vi "Register Disabled Save.vi"(8 "error in (no error)":errorcluster, 11 "UI Controller in":refnum<class "UI Controller.lvclass">) -> (0 "error out":errorcluster, 3 "UI Controller out":refnum<class "UI Controller.lvclass">)   [LabVIEW 2020, in "UI Controller.lvlib" / "UI Controller.lvclass"]
uses:
  UI Controller.lvclass
  C:/Program Files/National Instruments/LabVIEW 2020/vi.lib/ActorFrameworkMVC/Abstract Controller/Abstract Controller/Abstract Controller.lvclass
  Models/Yaml Model/Yaml Model Messages/Register Disabled Save Msg/Register Disabled Save Msg.lvclass
  C:/Program Files/National Instruments/LabVIEW 2020/vi.lib/ActorFramework/Message/Message.lvclass
  Views/Side Menu View/Side Menu View Messages/Concrete Disabled Save Msg/Concrete Disabled Save Msg.lvclass
  C:/Program Files/National Instruments/LabVIEW 2020/vi.lib/ActorFrameworkObserver/Data Message/Data Message.lvclass
  <vilib>/ActorFramework/Message Enqueuer/Message Enqueuer.lvclass/Message Enqueuer.ctl
  Models/Map Model/Map Model Messages/Register Disabled Save Msg/Register Disabled Save Msg.lvclass
  <vilib>/ActorFramework/Message Priority Queue/Priority Enqueue.vi
  <vilib>/ActorFrameworkMVC/Abstract Controller/Abstract Controller/Abstract Controller.lvclass
  <vilib>/ActorFramework/Message Enqueuer/Message Enqueuer.lvclass
panel:
  # "NOTICE -- YOU MUST LEAVE THIS NOTICE IN PLACE.\n\nCopyright (c) 2017, LIANG LIU Shawn.Liu.cn@gmail.com\nAll rights reserved.\n\nRedistribution and use in source and binary forms, with or without modification, are permitted provided that the following conditions are met:\n-Redistributions of source code must retain the above copyright notice, this list of conditions and the following disclaimer.\n-Redistributions in binary form must reproduce the above copyright notice, this list of conditions and the following disclaimer in the documentation and/or other materials provided with the distribution.\n-Neither the name of the eLp nor the names of its contributors may be used to endorse or promote products derived from this software without specific prior written permission.\n\nTHIS SOFTWARE IS PROVIDED BY THE COPYRIGHT HOLDERS AND CONTRIBUTORS \"AS IS\" AND ANY EXPRESS OR IMPLIED WARRANTIES, INCLUDING, BUT NOT LIMITED TO, THE IMPLIED WARRANTIES OF MERCHANTABILITY AND FITNESS FOR A PARTICULAR PURPOSE ARE DISCLAIMED. IN NO EVENT SHALL THE COPYRIGHT HOLDER OR CONTRIBUTORS BE LIABLE FOR ANY DIRECT, INDIRECT, INCIDENTAL, SPECIAL, EXEMPLARY, OR CONSEQUENTIAL DAMAGES (INCLUDING, BUT NOT LIMITED TO, PROCUREMENT OF SUBSTITUTE GOODS OR SERVICES; LOSS OF USE, DATA, OR PROFITS; OR BUSINESS INTERRUPTION) HOWEVER CAUSED AND ON ANY THEORY OF LIABILITY, WHETHER IN CONTRACT, STRICT LIABILITY, OR TORT (INCLUDING NEGLIGENCE OR OTHERWISE) ARISING IN ANY WAY OUT OF THE USE OF THIS SOFTWARE, EVEN IF ADVISED OF THE POSSIBILITY OF SUCH DAMAGE."
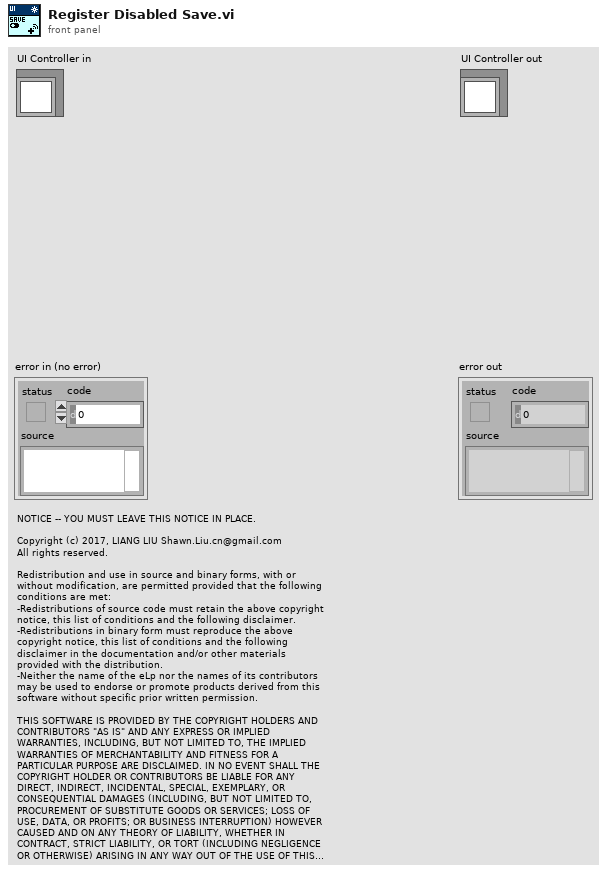
[diagram p1: front panel]
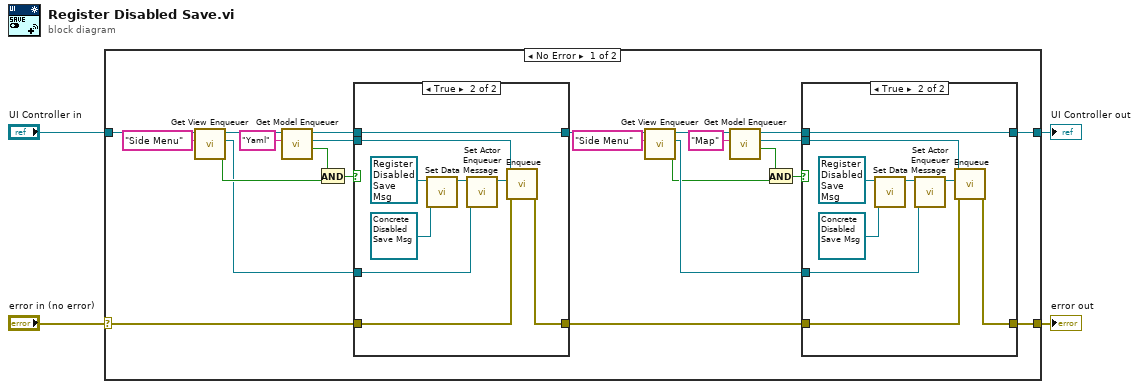
[diagram p0: block diagram]
diagram:
  n1 = case shown="No Error" "error in (no error)" {
    selector: "error in (no error)" -> [w27 w52]
    tunnel: "UI Controller in" -> [w28 w51]
    tunnel: [w26 w51] -> w2
    tunnel: [w25 w52] -> w1
    frame No Error {
      n2 = call <vilib>:"Get View Enqueuer.vi"("View Name"="Side Menu" ("Model Name"), "Abstract Controller in"=w28) -> ("Found?"=w17:bool, "View Enqueuer"=w16:refnum<class "Message Enqueuer.lvclass">, "Abstract Controller out"=w21:refnum<class "UI Controller.lvclass">)  [unwired: 6 in, 1 out]
      n3 = call <vilib>:"Get Model Enqueuer.vi"("Model Name"="Yaml" ("View Name"), "Abstract Controller in"=w21) -> ("Found?"=w18:bool, "Model Enqueuer"=w23:refnum<class "Message Enqueuer.lvclass">, "Abstract Controller out"=w22:refnum<class "UI Controller.lvclass">)  [unwired: 6 in, 1 out]
      n4 = And(x=w18, y=w17) -> (x .and. y?=w19:bool)
      n5 = case shown="True" w19 {
        tunnel: w23 -> [_ w46]
        tunnel: w22 -> [w41 w47]
        tunnel: [w41 w47] -> w6
        tunnel: w27 -> [w40 w44]
        tunnel: [w40 w43] -> w5
        tunnel: w16 -> [_ w42]
        frame False {
        }
        frame True {
          n6 = call-dynamic "Set Data Message.vi"("Data Message"=refnum<class "Concrete Disabled Save Msg.lvclass"> refnum ("Side Menu View.lvlib:Concrete Disabled Save Msg.lvclass"), "Registration Message in"=refnum<class "Register Disabled Save Msg.lvclass"> refnum ("Yaml Model.lvlib:Register Disabled Save Msg.lvclass")) -> ("Registration Message out"=w49:refnum<class "Register Disabled Save Msg.lvclass">)  [unwired: 9 in]
          n7 = call-dynamic "Set Actor Enqueuer.vi"("Actor Enqueuer"=w42, "Registration Message in"=w49) -> ("Registration Message out"=w45:refnum<class "Register Disabled Save Msg.lvclass">)  [unwired: 9 in]
          n8 = call <vilib>:"Enqueue.vi"("error in (no error)"=w44, "Message"=w45, "Message Enqueuer in"=w46) -> ("error out"=w43:errorcluster)  [unwired: 7 in, 1 out]
        }
      }
      n9 = call <vilib>:"Get View Enqueuer.vi"("View Name"="Side Menu" ("Model Name"), "Abstract Controller in"=w6) -> ("Found?"=w14:bool, "View Enqueuer"=w15:refnum<class "Message Enqueuer.lvclass">, "Abstract Controller out"=w10:refnum<class "UI Controller.lvclass">)  [unwired: 6 in, 1 out]
      n10 = call <vilib>:"Get Model Enqueuer.vi"("Model Name"="Map" ("View Name"), "Abstract Controller in"=w10) -> ("Found?"=w13:bool, "Model Enqueuer"=w8:refnum<class "Message Enqueuer.lvclass">, "Abstract Controller out"=w9:refnum<class "UI Controller.lvclass">)  [unwired: 6 in, 1 out]
      n11 = And(x=w13, y=w14) -> (x .and. y?=w12:bool)
      n12 = case shown="True" w12 {
        tunnel: w8 -> [_ w35]
        tunnel: w9 -> [w30 w36]
        tunnel: [w30 w36] -> w26
        tunnel: w5 -> [w29 w33]
        tunnel: [w29 w32] -> w25
        tunnel: w15 -> [_ w31]
        frame False {
        }
        frame True {
          n13 = call-dynamic "Set Data Message.vi"("Data Message"=refnum<class "Concrete Disabled Save Msg.lvclass"> refnum ("Side Menu View.lvlib:Concrete Disabled Save Msg.lvclass"), "Registration Message in"=refnum<class "Register Disabled Save Msg.lvclass"> refnum ("Map Model.lvlib:Register Disabled Save Msg.lvclass")) -> ("Registration Message out"=w38:refnum<class "Register Disabled Save Msg.lvclass">)  [unwired: 9 in]
          n14 = call-dynamic "Set Actor Enqueuer.vi"("Actor Enqueuer"=w31, "Registration Message in"=w38) -> ("Registration Message out"=w34:refnum<class "Register Disabled Save Msg.lvclass">)  [unwired: 9 in]
          n15 = call <vilib>:"Enqueue.vi"("error in (no error)"=w33, "Message"=w34, "Message Enqueuer in"=w35) -> ("error out"=w32:errorcluster)  [unwired: 7 in, 1 out]
        }
      }
    }
    frame Error {
    }
  }
  "error out" <- w1
  "UI Controller out" <- w2
